vi "Simple Y16 IMAQ.vi"() -> ()   [LabVIEW 2010]
panel:
  in  "stop":bool
  out "Image":T1(plugin-control)
  out "Error Out":errorcluster
  in  "ICImagingControl":refnum<k7>(container)
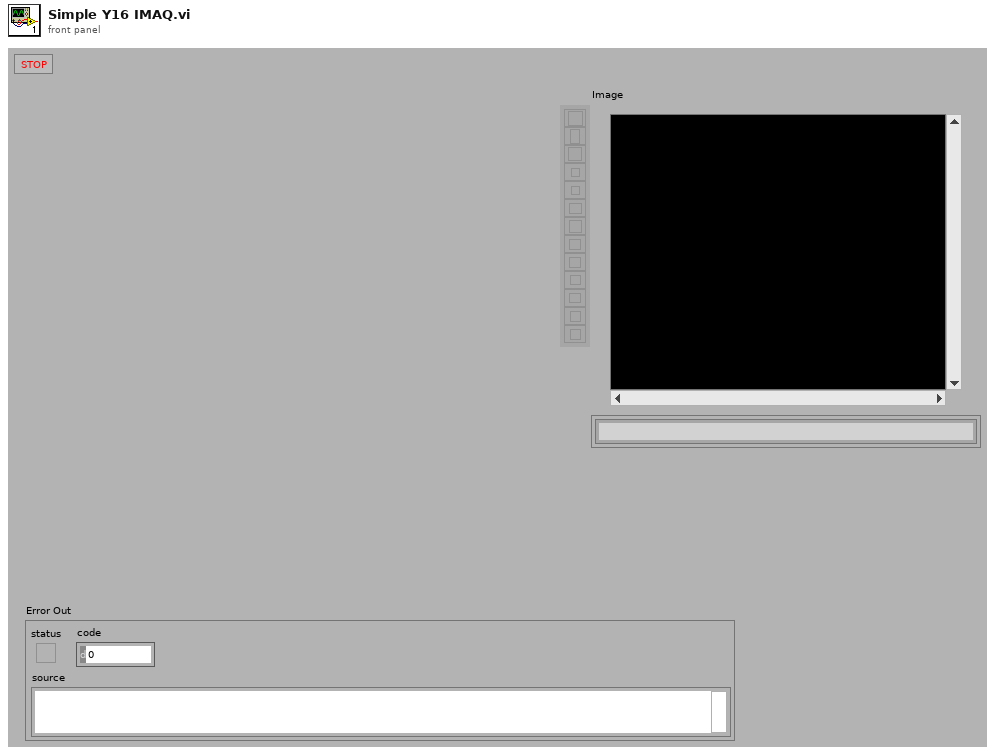
[diagram p1: front panel]
types:
  T1 = typedef "IMAQ Image.ctl" = refnum<image>
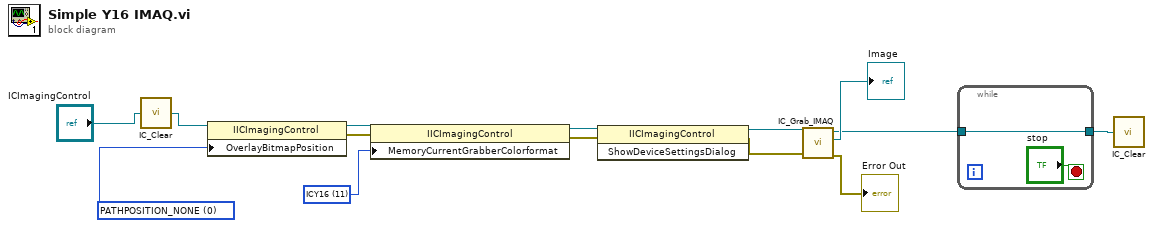
[diagram p0: block diagram]
diagram:
  w14 = 0 items=["PATHPOSITION_NONE"=0, "PATHPOSITION_DEVICE"=1, "PATHPOSITION_SINK"=2, "PATHPOSITION_DISPLAY"=4] ("OverlayBitmapPosition")
  w13 = 11 items=["ICRGB32"=1, "ICRGB24"=2, "ICRGB565"=3, "ICRGB555"=4, "ICY8"=5, "ICUYVY"=6, "ICY800"=7, "ICYGB1"=8, "ICYGB0"=9, "ICBY8"=10, "ICY16"=11] ("MemoryCurrentGrabberColorformat")
  n1 = call "IC_Clear.vi"("ICImagingControl 2"="ICImagingControl") -> ("ICImagingControl"=w11:refnum<k7>)
  n2 = property class="IICImagingControl"(reference=w11, "OverlayBitmapPosition"=w14) -> (reference out=w10:refnum<k7>, error out=w8:errorcluster)  [unwired: 1 in]
  n3 = property class="IICImagingControl"(reference=w10, error in=w8, "MemoryCurrentGrabberColorformat"=w13) -> (reference out=w9:refnum<k7>, error out=w7:errorcluster)
  n4 = invoke class="IICImagingControl" method="ShowDeviceSettingsDialog"(reference=w9, error in=w7) -> (reference out=w6:refnum<k7>, error out=w5:errorcluster)  [unwired: 1 in, 1 out]
  n5 = call "IC_Grab_IMAQ.vi"("ICImagingControl In"=w6, "Error In (no error)"=w5) -> ("ICImagingControl Out"=w2:refnum<k7>, "Image Out"=→"Image":T1, "Error Out"=→"Error Out":errorcluster)  [unwired: 1 in, 1 out]
  n6 = while {
    tunnel: w2 -> [w15]
    tunnel: [w15] -> w1
    stop <- "stop" stop-if-true
  }
  n7 = call "IC_Clear.vi"("ICImagingControl 2"=w1) -> ()  [unwired: 1 out]
